vi "Main.vi"(10 "DAQ Type":enum16{"Hardware", "Simulation"}(ring), 11 "Module Admin":refnum<class "Delacor_lib_QMH_Module Admin.lvclass">) -> ()   [LabVIEW 2021, in "CVT.lvlib"]
doc: "This template is based off of the Queued Message Handler design pattern and the Queued Message Handler project template that ships with LabVIEW.\n\nThe main difference is that the queue is private to this module and communication between modules is performed via Broadcast and Request events.\n\nRequest events are wrapped in public API methods and are handled in the Event Handling Loop (EHL) of this VI. Any module can register for Broadcast events sent by this module. The EHL generates messages based on user interface actions.\n\nThe Message Handling Loop (MHL) processes messages generated by the EHL, or by other messages. The messages are string values, so new messages can be added easily to the Message Cases case structure in the MHL. Each message cluster can also provide an optional value for Message Data, which is a variant that can be converted to whatever message-specific data is required.\n_____\nBased on DQMH Project Template 6.1.0.94."
uses:
  CVT.lvlib
  <vilib>/Delacor/Delacor QMH/Libraries/Module Admin_class/Delacor_lib_QMH_Module Admin.lvclass
  <vilib>/NI/Current Value Table/Type Defs/File Format.ctl
  <vilib>/NI/Current Value Table/Type Defs/Single Tag.ctl
  <vilib>/NI/Current Value Table/Type Defs/Data Types.ctl
  <vilib>/NI/Current Value Table/Type Defs/Tag Grouping set.ctl
  Module Data--cluster.ctl
  <vilib>/Delacor/Delacor QMH/Libraries/Message Queue_class/Delacor_lib_QMH_Message Queue.lvclass/Delacor_lib_QMH_Message Queue.ctl
  Stop Argument--cluster.ctl
  <vilib>/Delacor/Delacor QMH/Libraries/Module Admin_class/Delacor_lib_QMH_Module Admin.lvclass/Delacor_lib_QMH_Module Admin.ctl
  REQ DC PWS Connect Argument--cluster.ctl
  Input Command.ctl
  REQ Write AO Data Argument--cluster.ctl
  <vilib>/Utility/miscctls.llb/LVPointTypeDef.ctl
  <vilib>/NI/Current Value Table/Type Defs/Group Data.ctl
  <vilib>/Delacor/Delacor QMH/Libraries/Message Queue_class/Delacor_lib_QMH_Enqueue Message (Single).vi
  <vilib>/Delacor/Delacor QMH/Libraries/Module Admin_class/Delacor_lib_QMH_Get External Launch.vi
  <vilib>/NI/Current Value Table/DataTypes/Boolean_Write.vi
  <vilib>/NI/Current Value Table/DataTypes/Double_Get Index.vi
  <vilib>/NI/Current Value Table/Type to Enum.vi
  <vilib>/NI/Current Value Table/DataTypes/Boolean_Type To Enum.vi
  <vilib>/NI/Current Value Table/DataTypes/Double_Type To Enum.vi
  <vilib>/NI/Current Value Table/Read tags into grouped data.vi
  <vilib>/NI/Current Value Table/Write grouped data to tags.vi
  <vilib>/NI/Current Value Table/Read Index Set.vi
  <vilib>/NI/Current Value Table/DataTypes/Double_Read Index Set.vi
  <vilib>/NI/Current Value Table/DataTypes/Array of String_Read Index Set.vi
  <vilib>/NI/Current Value Table/DataTypes/Array of Boolean_Read Index Set.vi
  <vilib>/NI/Current Value Table/DataTypes/Array of Single_Read Index Set.vi
  <vilib>/NI/Current Value Table/DataTypes/Array of Double_Read Index Set.vi
  <vilib>/NI/Current Value Table/DataTypes/Array of I8_Read Index Set.vi
  <vilib>/NI/Current Value Table/DataTypes/Array of I16_Read Index Set.vi
  <vilib>/NI/Current Value Table/DataTypes/Array of I32_Read Index Set.vi
  <vilib>/NI/Current Value Table/DataTypes/Array of I64_Read Index Set.vi
  <vilib>/NI/Current Value Table/DataTypes/Array of U64_Read Index Set.vi
  <vilib>/NI/Current Value Table/DataTypes/Array of U32_Read Index Set.vi
  <vilib>/NI/Current Value Table/DataTypes/Array of U16_Read Index Set.vi
  <vilib>/NI/Current Value Table/DataTypes/Array of U8_Read Index Set.vi
  <vilib>/NI/Current Value Table/DataTypes/Boolean_Read Index Set.vi
  <vilib>/NI/Current Value Table/DataTypes/String_Read Index Set.vi
  <vilib>/NI/Current Value Table/DataTypes/U8_Read Index Set.vi
  <vilib>/NI/Current Value Table/DataTypes/U16_Read Index Set.vi
  <vilib>/NI/Current Value Table/DataTypes/U32_Read Index Set.vi
  <vilib>/NI/Current Value Table/DataTypes/U64_Read Index Set.vi
  <vilib>/NI/Current Value Table/DataTypes/I8_Read Index Set.vi
  <vilib>/NI/Current Value Table/DataTypes/I16_Read Index Set.vi
  <vilib>/NI/Current Value Table/DataTypes/I32_Read Index Set.vi
  <vilib>/NI/Current Value Table/DataTypes/I64_Read Index Set.vi
  <vilib>/NI/Current Value Table/DataTypes/Single_Read Index Set.vi
  <vilib>/NI/Current Value Table/Write Index Set.vi
  <vilib>/NI/Current Value Table/DataTypes/Double_Write Index Set.vi
  <vilib>/NI/Current Value Table/DataTypes/Array of String_Write Index Set.vi
  <vilib>/NI/Current Value Table/DataTypes/Array of Boolean_Write Index Set.vi
  <vilib>/NI/Current Value Table/DataTypes/Array of Single_Write Index Set.vi
  <vilib>/NI/Current Value Table/DataTypes/Array of Double_Write Index Set.vi
  <vilib>/NI/Current Value Table/DataTypes/Array of I8_Write Index Set.vi
  <vilib>/NI/Current Value Table/DataTypes/Array of I16_Write Index Set.vi
  <vilib>/NI/Current Value Table/DataTypes/Array of I32_Write Index Set.vi
  <vilib>/NI/Current Value Table/DataTypes/Array of I64_Write Index Set.vi
  <vilib>/NI/Current Value Table/DataTypes/Array of U64_Write Index Set.vi
  <vilib>/NI/Current Value Table/DataTypes/Array of U32_Write Index Set.vi
  <vilib>/NI/Current Value Table/DataTypes/Array of U16_Write Index Set.vi
  <vilib>/NI/Current Value Table/DataTypes/Array of U8_Write Index Set.vi
  <vilib>/NI/Current Value Table/DataTypes/Boolean_Write Index Set.vi
  <vilib>/NI/Current Value Table/DataTypes/String_Write Index Set.vi
  <vilib>/NI/Current Value Table/DataTypes/U8_Write Index Set.vi
  <vilib>/NI/Current Value Table/DataTypes/U16_Write Index Set.vi
  <vilib>/NI/Current Value Table/DataTypes/U32_Write Index Set.vi
  <vilib>/NI/Current Value Table/DataTypes/U64_Write Index Set.vi
  <vilib>/NI/Current Value Table/DataTypes/I8_Write Index Set.vi
  <vilib>/NI/Current Value Table/DataTypes/I16_Write Index Set.vi
  <vilib>/NI/Current Value Table/DataTypes/I32_Write Index Set.vi
  <vilib>/NI/Current Value Table/DataTypes/I64_Write Index Set.vi
  <vilib>/NI/Current Value Table/DataTypes/Single_Write Index Set.vi
  <vilib>/Utility/error.llb/Error Cluster From Error Code.vi
  <vilib>/NI/Current Value Table/FGVs/CVT Globals.vi
  <vilib>/NI/Current Value Table/FGVs/Tag Memory.vi
  <vilib>/NI/Current Value Table/Memory Block.vi
  <vilib>/NI/Current Value Table/DataTypes/Boolean_Memory Block.vi
  <vilib>/NI/Current Value Table/FGVs/Group Memory.vi
  <vilib>/NI/Current Value Table/DataTypes/Double_Memory Block.vi
  <vilib>/NI/Current Value Table/DataTypes/Array of String_Memory Block.vi
  <vilib>/NI/Current Value Table/DataTypes/Array of Boolean_Memory Block.vi
  <vilib>/NI/Current Value Table/DataTypes/Array of Single_Memory Block.vi
  <vilib>/NI/Current Value Table/DataTypes/Array of Double_Memory Block.vi
  <vilib>/NI/Current Value Table/DataTypes/Array of I8_Memory Block.vi
  <vilib>/NI/Current Value Table/DataTypes/Array of I16_Memory Block.vi
  <vilib>/NI/Current Value Table/DataTypes/Array of I32_Memory Block.vi
  <vilib>/NI/Current Value Table/DataTypes/Array of I64_Memory Block.vi
  <vilib>/NI/Current Value Table/DataTypes/Array of U64_Memory Block.vi
  <vilib>/NI/Current Value Table/DataTypes/Array of U32_Memory Block.vi
  <vilib>/NI/Current Value Table/DataTypes/Array of U16_Memory Block.vi
  <vilib>/NI/Current Value Table/DataTypes/Array of U8_Memory Block.vi
  <vilib>/NI/Current Value Table/DataTypes/String_Memory Block.vi
  <vilib>/NI/Current Value Table/DataTypes/U8_Memory Block.vi
  <vilib>/NI/Current Value Table/DataTypes/U16_Memory Block.vi
  <vilib>/NI/Current Value Table/DataTypes/U32_Memory Block.vi
  <vilib>/NI/Current Value Table/DataTypes/U64_Memory Block.vi
  <vilib>/NI/Current Value Table/DataTypes/I8_Memory Block.vi
  <vilib>/NI/Current Value Table/DataTypes/I16_Memory Block.vi
  <vilib>/NI/Current Value Table/DataTypes/I32_Memory Block.vi
  <vilib>/NI/Current Value Table/DataTypes/I64_Memory Block.vi
  <vilib>/NI/Current Value Table/DataTypes/Single_Memory Block.vi
  <vilib>/ErrorRing/Error Ring.xnode
  <vilib>/Delacor/Delacor QMH/Libraries/Message Queue_class/Delacor_lib_QMH_Message Queue.lvclass
  DAQ Hardware/DAQ Hardware.lvlib
  Error Log/Error Log.lvlib
  <vilib>/NI/Current Value Table/Current Value Table.lvlib
panel:
  out "CVT Tags to Create Out":T1
  in  "CVT Tags to Create":T1
  out "error out":errorcluster
  out "Status":string
  in  "Simulate MHL Error":bool
  in  "Simulate EHL Error":bool
  # "Other QMH Modules communicate with this Module via its Public API (wrappers for its Request Events).\n\nThis Module communicates with other Modules via its Broadcast Events.\nAny module that wants to get these messages, just registers for this module's Broadcast events."
  # "This template is for the Delacor Modified Queued Message Handler design pattern.\n\nSee the block diagram for more information on how to use this template."
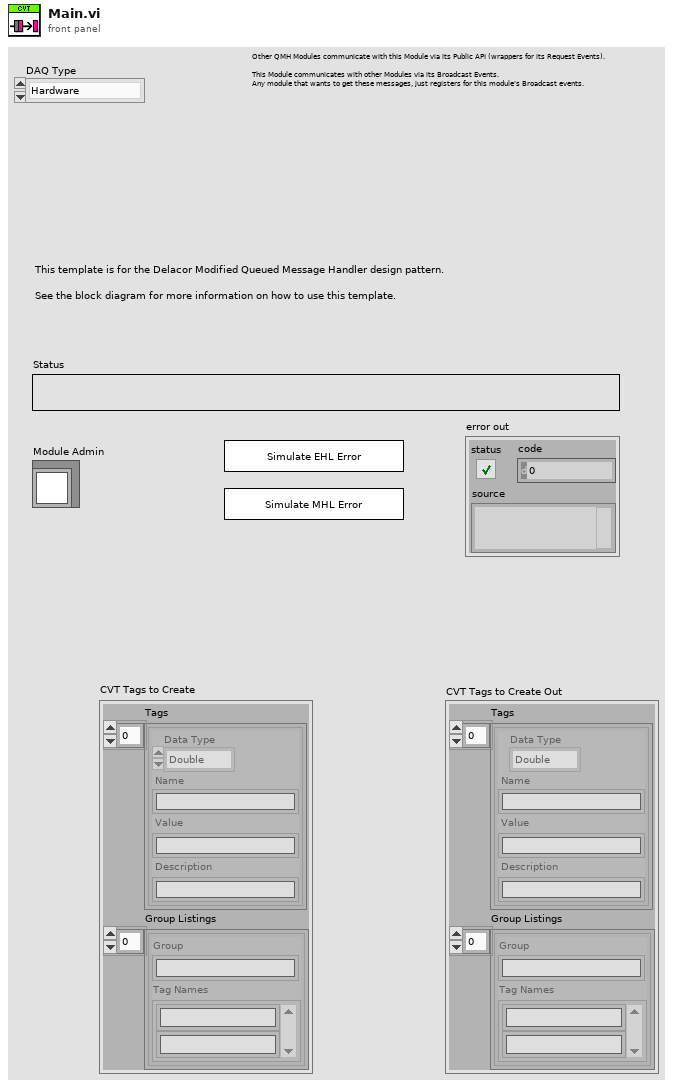
[diagram p1: front panel]
types:
  T1 = typedef "Current Value Table.lvlib/File Format.ctl" = cluster{"Tags":T2[], "Group Listings":T4[]}
  T2 = typedef "Current Value Table.lvlib/Single Tag.ctl" = cluster{"Data Type":T3, "Name":string, "Value":string, "Description":string}
  T3 = typedef "Current Value Table.lvlib/Data Types.ctl" = enum16{"Double", "Single", "I64", "I32", "I16", "I8", "U64", "U32", "U16", "U8", "String", "Boolean", "Array of U8", "Array of U16", "Array of U32", "Array of U64", "Array of I64", "Array of I32", "Array of I16", "Array of I8", "Array of Double", "Array of Single", "Array of Boolean", "Array of String"}
  T4 = typedef "Current Value Table.lvlib/Tag Grouping set.ctl" = cluster{"Group":string, "Tag Names":string[]}
  T5 = typedef "CVT.lvlib/Request Events--cluster.ctl" = cluster{"Stop Module":refnum<user-event>, "Show Panel":refnum<user-event>, "Hide Panel":refnum<user-event>, "Get Module Execution Status":refnum<user-event>, "Show Diagram":refnum<user-event>, "REQ DC PWS Connect":refnum<user-event>, "REQ Write AO Data":refnum<user-event>}
  T6 = typedef "CVT.lvlib/Module Data--cluster.ctl" = cluster{"Status":string}
  T7 = enum32{"invalid lock state", "Not Locked", "Locked (No Password)", "Password-protected"}
  T8 = typedef "CVT.lvlib/Stop Argument--cluster.ctl" = cluster{"Origin":string, "Exit via Stop Module Req?":bool, "Wait for Module to stop?":bool}
  T9 = typedef "CVT.lvlib/REQ DC PWS Connect Argument--cluster.ctl" = cluster{"Connect ?":bool, "Command":T10}
  T10 = typedef "CVT.lvlib/Input Command.ctl" = enum16{"DC PWS", "DMM", "FGEN", "Oscill", "NI DAQ", "NI DIO", "NI CAN", "ESPEC", "ARINC", "MATRIX"}
  T11 = typedef "CVT.lvlib/REQ Write AO Data Argument--cluster.ctl" = cluster{"AO Name":string, "Data":dbl}
  T12 = typedef "LVPointTypeDef.ctl" = cluster{"Horizontal":i16, "Vertical":i16}
  T13 = enum32{"Invalid", "Standard", "Closed", "Hidden", "Minimized", "Maximized"}
  T14 = typedef "Current Value Table.lvlib/Group Data.ctl" = cluster{"Double":dbl[], "Single":sgl[], "I64":i64[], "I32":i32[], "I16":i16[], "I8":i8[], "U64":u64[], "U32":u32[], "U16":u16[], "U8":u8[], "String":string[], "Boolean":bool[], "Array of U8":cluster{"U8 Array":u8[]}[], "Array of U16":cluster{"U16 Array":u16[]}[], "Array of U32":cluster{"U32 Array":u32[]}[], "Array of U64":cluster{"U64 Array":u64[]}[], "Array of I64":cluster{"I64 Array":i64[]}[], "Array of I32":cluster{"I32 Array":i32[]}[], "Array of I16":cluster{"I16 Array":i16[]}[], "Array of I8":cluster{"I8 Array":i8[]}[], "Array of Double":cluster{"DBL Array":dbl[]}[], "Array of Single":cluster{"SGL Array":sgl[]}[], "Array of Boolean":cluster{"Boolean Array":bool[]}[], "Array of String":cluster{"String Array":string[]}[]}
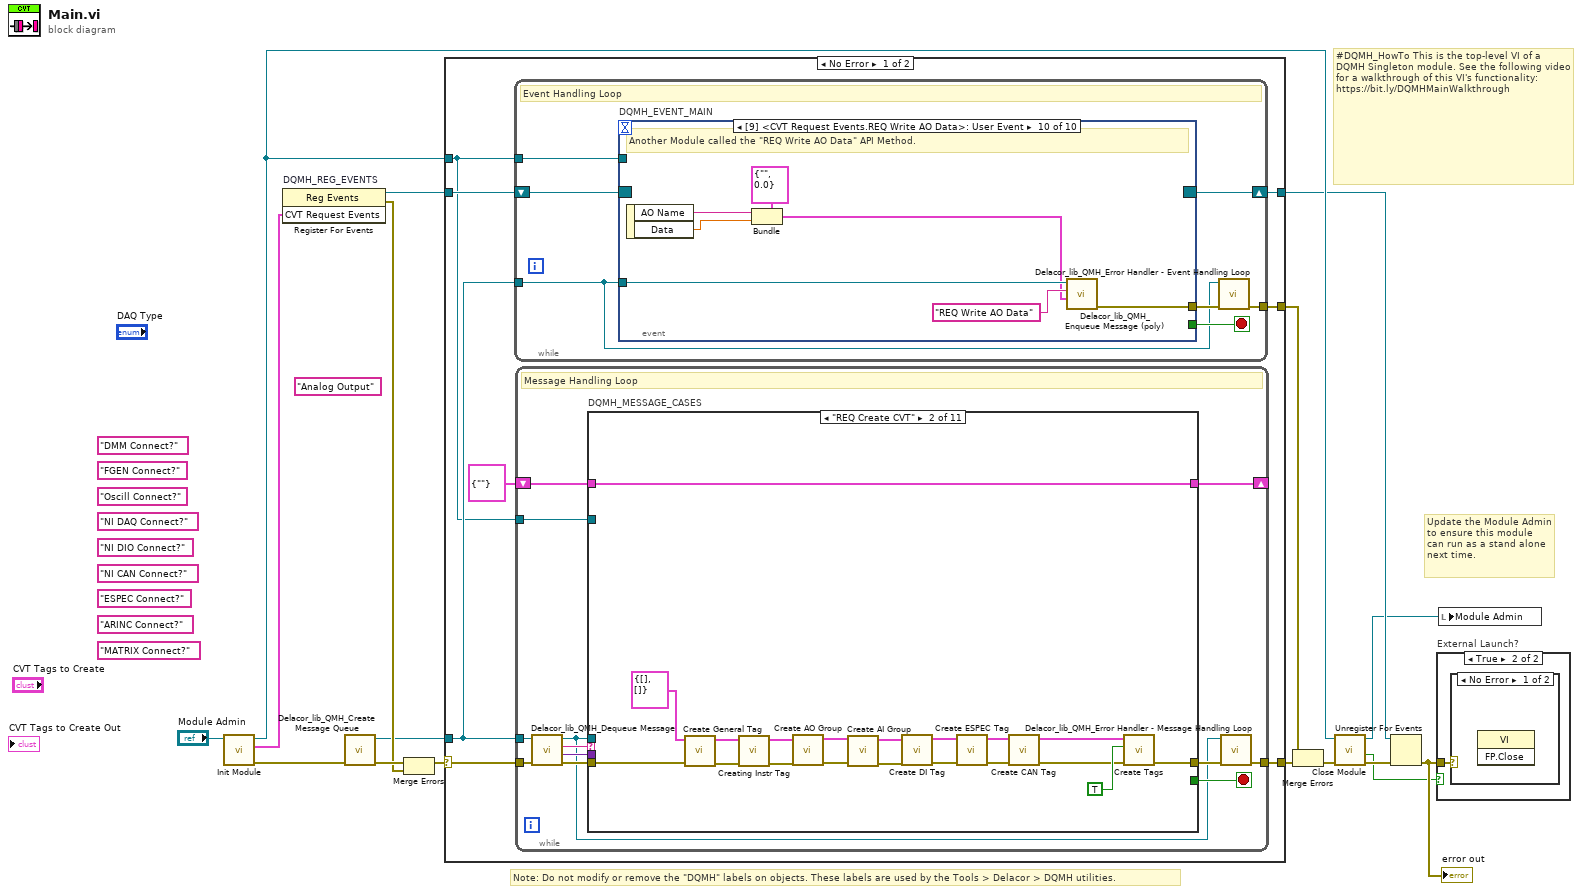
[diagram p0: block diagram]
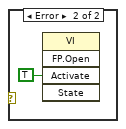
[diagram p3: hidden frame]
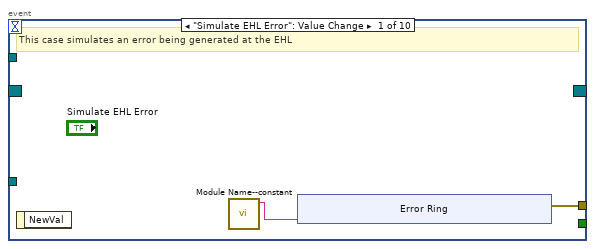
[diagram p4: hidden frame]
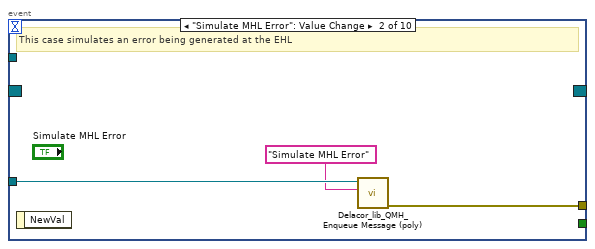
[diagram p5: hidden frame]
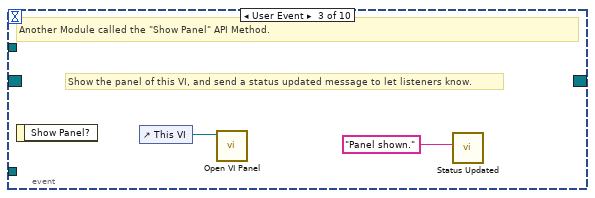
[diagram p6: hidden frame]
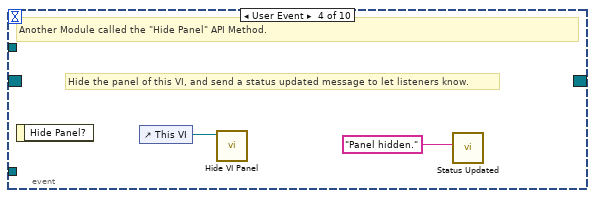
[diagram p7: hidden frame]
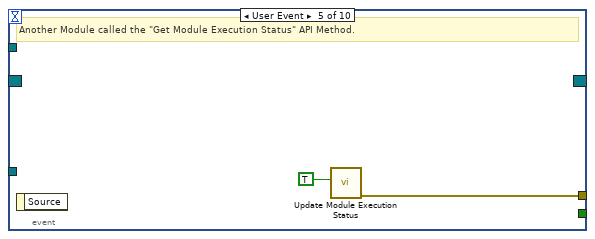
[diagram p8: hidden frame]
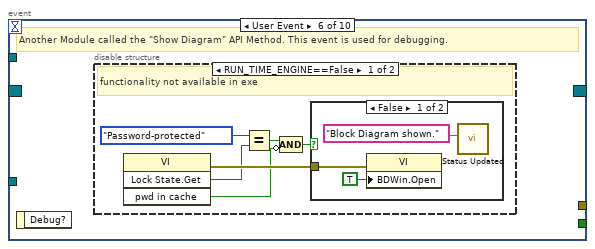
[diagram p9: hidden frame]
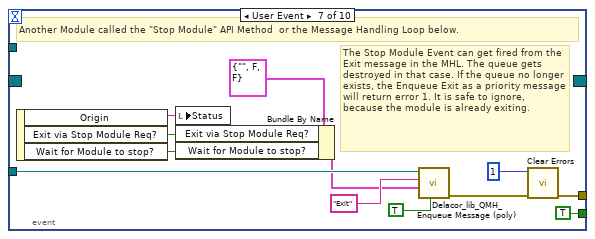
[diagram p12: hidden frame]
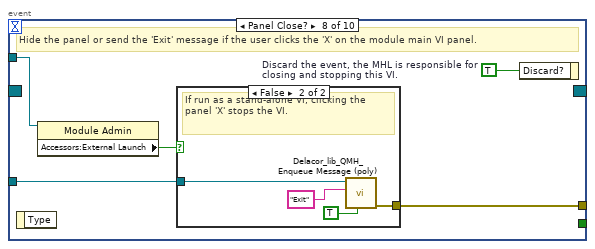
[diagram p13: hidden frame]
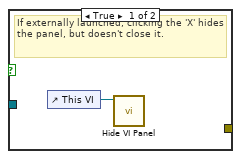
[diagram p14: hidden frame]
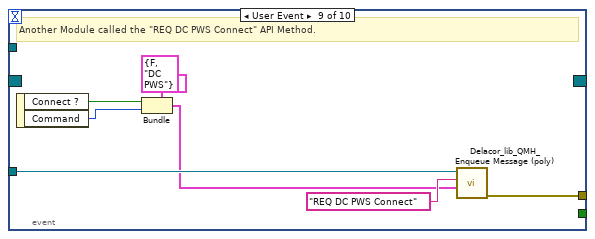
[diagram p15: hidden frame]
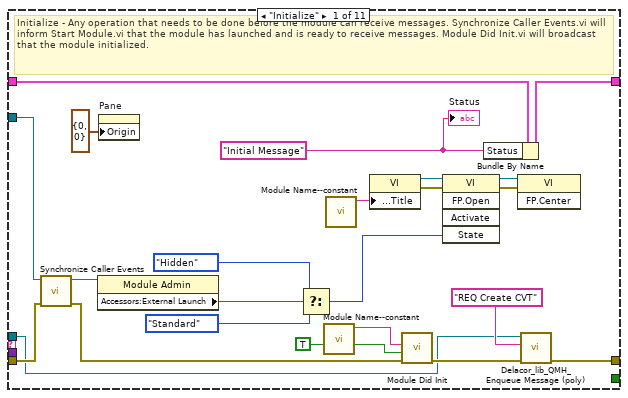
[diagram p16: hidden frame]
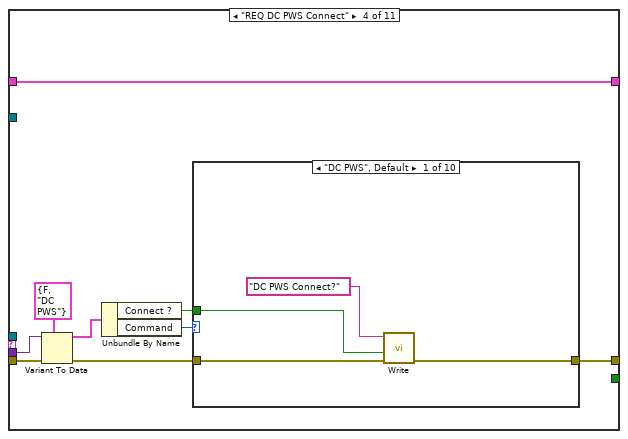
[diagram p18: hidden frame]
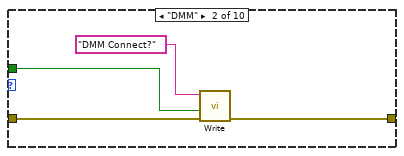
[diagram p19: hidden frame]
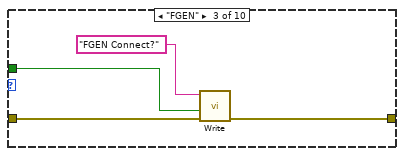
[diagram p20: hidden frame]
diagram:
  (unwired) "Analog Output" ("Group")
  (unwired) "MATRIX Connect?" ("Tag Name")
  (unwired) "ARINC Connect?" ("Tag Name")
  (unwired) "ESPEC Connect?" ("Tag Name")
  (unwired) "NI CAN Connect?" ("Tag Name")
  (unwired) "NI DIO Connect?" ("Tag Name")
  (unwired) "NI DAQ Connect?" ("Tag Name")
  (unwired) "Oscill Connect?" ("Tag Name")
  (unwired) "FGEN Connect?" ("Tag Name")
  (unwired) "DMM Connect?" ("Tag Name")
  # "#DQMH_HowTo This is the top-level VI of a DQMH Singleton module. See the following video for a walkthrough of this VI's functionality: https://bit.ly/DQMHMainWalkthrough"
  # "Note: Do not modify or remove the \"DQMH\" labels on objects. These labels are used by the Tools > Delacor > DQMH utilities."
  # "Update the Module Admin to ensure this module can run as a stand alone next time."
  n1 = call "Init Module.vi"("Singleton Module Admin in"="Module Admin") -> ("error out"=w16:errorcluster, "CVT Request Events"=w5:T5, "Singleton Module Admin out"=w8:refnum<class "Delacor_lib_QMH_Module Admin.lvclass">)  [unwired: 8 in]
  n2 = register-events "DQMH_REG_EVENTS"(w5) -> (reference out=w6:refnum<event-registration>, error out=w9:errorcluster)  [unwired: 2 in]
  n3 = call <vilib>:"Delacor_lib_QMH_Create Message Queue.vi"("error in"=w16) -> ("error out"=w11:errorcluster, "Message Queue"=w4:refnum<class "Delacor_lib_QMH_Message Queue.lvclass">)  [unwired: 9 in]
  n4 = Merge Errors(w11, w9) -> (w10:errorcluster)
  n5 = case shown="No Error" w10 {
    selector: w10 -> [w23 w286]
    tunnel: [w25 w285] -> w17
    tunnel: [w22 w291] -> w7
    tunnel: w6 -> [w20 w291]
    tunnel: w4 -> [w19 w284]
    tunnel: [w24 _] -> w14
    tunnel: w8 -> [w18 w287]
    frame No Error {
      n6 = while {
        tunnel: w19 -> [w26]
        shift-right: [w29] -> w22
        shift-left: w20 -> [w30]
        tunnel: [w31] -> w24
        tunnel: w18 -> [w27]
        stop <- w28 stop-if-true
        # "Event Handling Loop"
        n7 = event "DQMH_EVENT_MAIN" shown="[9] <CVT Request Events.REQ Write AO Data>: User Event" {
          selector: w30 -> [_ _ _ _ _ _ _ _ _ _]
          dyn-events: [_ _ _ _ _ _ _ _ _ _] -> w29
          timeout: _ -> [_ _ _ _ _ _ _ _ _ _]
          tunnel: [_ _ _ _ _ _ TRUE ("Discard?") _ _ _] -> w28
          tunnel: w26 -> [_ w43 _ _ _ _ w67 w74 w88 w95]
          tunnel: [w34 w44 _ _ w50 _ w70 w76 w83 w91] -> w32
          tunnel: w27 -> [_ _ _ _ _ _ _ w73 _ _]
          event "Simulate EHL Error": Value Change {
            # "This case simulates an error being generated at the EHL"
            n8 = event-data() -> ()  [unwired: 1 in, 1 out]
            n9 = call "Module Name--constant.vi"() -> ("Module Name"=w33:string)  [unwired: 11 in]
            n10 = xnode "Error Ring"("parameter 0"=w33) -> ("error out"=w34:errorcluster)
          }
          event "Simulate MHL Error": Value Change {
            # "This case simulates an error being generated at the EHL"
            n11 = event-data() -> ()  [unwired: 1 in, 1 out]
            n12 = call-poly <vilib>:"Delacor_lib_QMH_Enqueue Message (poly).vi"("Message"="Simulate MHL Error", "Message Queue in"=w43) -> ("error out"=w44:errorcluster)  [unwired: 8 in, 1 out]
          }
          event User Event {
            # "Show the panel of this VI, and send a status updated message to let listeners know."
            # "Another Module called the \"Show Panel\" API Method."
            n13 = event-data() -> ()  [unwired: 1 in, 1 out]
            n14 = control-ref of="This VI"() -> (w46:refnum<vi>)
            n15 = call "Open VI Panel.vi"("VI"=w46) -> ()  [unwired: 10 in, 1 out]
            n16 = call "Status Updated.vi"("Status"="Panel shown." ("format string")) -> ()  [unwired: 10 in, 1 out]
          }
          event User Event {
            # "Hide the panel of this VI, and send a status updated message to let listeners know."
            # "Another Module called the \"Hide Panel\" API Method."
            n17 = event-data() -> ()  [unwired: 1 in, 1 out]
            n18 = control-ref of="This VI"() -> (w48:refnum<vi>)
            n19 = call "Hide VI Panel.vi"("VI"=w48) -> ()  [unwired: 10 in, 1 out]
            n20 = call "Status Updated.vi"("Status"="Panel hidden." ("format string")) -> ()  [unwired: 10 in, 1 out]
          }
          event User Event {
            # "Another Module called the \"Get Module Execution Status\" API Method."
            n21 = event-data() -> ()  [unwired: 1 in, 1 out]
            n22 = call "Update Module Execution Status.vi"("Running?"=TRUE) -> ("error out"=w50:errorcluster)  [unwired: 10 in]
          }
          event User Event {
            # "Another Module called the \"Show Diagram\" API Method. This event is used for debugging."
            n23 = event-data() -> ()  [unwired: 1 in, 1 out]
            n24 = disable-structure shown="RUN_TIME_ENGINE==False" {
              frame condition #0 (active) {
                # "functionality not available in exe"
                n25 = invoke class="VI" method="Lock State.Get"() -> (error out=w56:errorcluster, "Get Lock State"=w55:T7, "pwd in cache"=w52:bool)  [unwired: 4 in, 1 out]
                n26 = Equal?(x=T7."Password-protected", y=w55) -> (x = y?=w53:bool)
                n27 = Compound Arithmetic op=AND(w53, invert w52) -> (w51:bool)
                n28 = case shown="False" w51 {
                  tunnel: w56 -> [w59 _]
                  frame False {
                    n29 = property class="VI"(error in=w59, "BDWin.Open"=TRUE ("Block Diagram Window:Open")) -> ()  [unwired: 1 in, 2 out]
                    n30 = call "Status Updated.vi"("Status"="Block Diagram shown." ("format string")) -> ()  [unwired: 10 in, 1 out]
                  }
                  frame True {
                    # "Password-protected VI, and the password is not in the cache. Do not show the diagram."
                  }
                }
              }
              frame condition #1 {
              }
            }
          }
          event User Event {
            # "The Stop Module Event can get fired from the Exit message in the MHL. The queue gets destroyed in that case. If the queue no longer exists, the Enqueue Exit as a priority message will return error 1. It is safe to ignore, because the module is already exiting."
            # "Another Module called the \"Stop Module\" API Method  or the Message Handling Loop below."
            n31 = event-data() -> ("Origin"=w66:string, "Exit via Stop Module Req?"=w62:bool, "Wait for Module to stop?"=w61:bool)  [unwired: 1 in]
            n32 = local write "Status"(w66) -> ()
            n33 = Bundle By Name(cluster=T8 {"Origin"="", "Exit via Stop Module Req?"=FALSE, "Wait for Module to stop?"=FALSE} ("Stop Argument"), "Exit via Stop Module Req?"=w62, "Wait for Module to stop?"=w61) -> (w60:T8)
            n34 = call-poly <vilib>:"Delacor_lib_QMH_Enqueue Message (poly).vi"("Priority Message? (F)"=TRUE, "Message Data"=w60, "Message"="Exit", "Message Queue in"=w67) -> ("error out"=w71:errorcluster)  [unwired: 6 in, 1 out]
            n35 = call <vilib>:"Clear Errors.vi"("error in (no error)"=w71, "specific error code to clear (0: all)"=1) -> ("error out"=w70:errorcluster)  [unwired: 4 in, 1 out]
          }
          event Panel Close? {
            w75 = TRUE  # Discard the event, the MHL is responsible for closing and stopping this VI.
            # "Hide the panel or send the 'Exit' message if the user clicks the 'X' on the module main VI panel."
            n36 = event-data() -> ()  [unwired: 1 in, 1 out]
            n37 = property class="Module Admin"(reference=w73) -> ("Accessors:External Launch"=w72:bool)  [unwired: 1 in, 2 out]
            n38 = case shown="False" w72 {
              tunnel: w74 -> [_ w80]
              tunnel: [_ w81] -> w76
              frame True {
                # "If externally launched, clicking the 'X' hides the panel, but doesn't close it."
                n39 = control-ref of="This VI"() -> (w77:refnum<vi>)
                n40 = call "Hide VI Panel.vi"("VI"=w77) -> ()  [unwired: 10 in, 1 out]
              }
              frame False {
                # "If run as a stand-alone VI, clicking the panel 'X' stops the VI."
                n41 = call-poly <vilib>:"Delacor_lib_QMH_Enqueue Message (poly).vi"("Priority Message? (F)"=TRUE, "Message"="Exit", "Message Queue in"=w80) -> ("error out"=w81:errorcluster)  [unwired: 7 in, 1 out]
              }
            }
            n42 = event-data("Discard?"=w75) -> ()  [unwired: 1 in, 1 out]
          }
          event User Event {
            # "Another Module called the \"REQ DC PWS Connect\" API Method."
            n43 = event-data() -> ("Connect ?"=w84:bool, "Command"=w82:T10)  [unwired: 1 in]
            n44 = Bundle(cluster=T9 {"Connect ?"=FALSE, "Command"=enum."DC PWS"} ("REQ DC PWS Connect Argument"), "Connect ?"=w84, "Command"=w82) -> (w85:T9)
            n45 = call-poly <vilib>:"Delacor_lib_QMH_Enqueue Message (poly).vi"("Message Data"=w85, "Message"="REQ DC PWS Connect", "Message Queue in"=w88) -> ("error out"=w83:errorcluster)  [unwired: 7 in, 1 out]
          }
          event User Event {
            # "Another Module called the \"REQ Write AO Data\" API Method."
            n46 = event-data() -> ("AO Name"=w90:string, "Data"=w89:dbl)  [unwired: 1 in]
            n47 = Bundle(cluster=T11 {"AO Name"="", "Data"=0.0} ("REQ Write AO Data Argument"), "AO Name"=w90, "Data"=w89) -> (w92:T11)
            n48 = call-poly <vilib>:"Delacor_lib_QMH_Enqueue Message (poly).vi"("Message Data"=w92, "Message"="REQ Write AO Data", "Message Queue in"=w95) -> ("error out"=w91:errorcluster)  [unwired: 7 in, 1 out]
          }
        }
        n49 = call-dynamic "Delacor_lib_QMH_Error Handler - Event Handling Loop.vi"("error in"=w32, "Message Queue in"=w26) -> ("dup error in"=w31:errorcluster)  [unwired: 8 in, 1 out]
      }
      n50 = while {
        tunnel: w19 -> [w98]
        shift-right: [w102] -> _
        shift-left: T6 {"Status"=""} ("Data Cluster") -> [w103]
        tunnel: w23 -> [w106]
        tunnel: [w104] -> w25
        tunnel: w18 -> [w96]
        stop <- w101 stop-if-true
        # "Message Handling Loop"
        n51 = call-dynamic "Delacor_lib_QMH_Dequeue Message.vi"("error in"=w106, "Message Queue in"=w98) -> ("error out"=w105:errorcluster, "Message Data"=w99:variant, "Message"=w100:string, "Message Queue out"=w97:refnum<class "Delacor_lib_QMH_Message Queue.lvclass">)  [unwired: 6 in]
        n52 = case "DQMH_MESSAGE_CASES" shown="\"REQ Create CVT\"" w100 {
          selector: w100 -> [_ _ _ _ _ _ _ _ _ _ w271]
          tunnel: w97 -> [w108 _ _ _ _ _ _ _ w241 w263 _]
          tunnel: w105 -> [w128 w142 w151 w160 w220 w223 w225 w230 w248 w269 w273]
          tunnel: [w109 w148 w151 w154 w216 w222 w225 w229 w244 w266 w274] -> w107
          tunnel: w103 -> [w118 w149 w150 w159 w219 w221 w224 w227 w243 w262 w272]
          tunnel: [w117 w149 w150 w159 w219 w221 w224 w227 w243 w262 w272] -> w102
          tunnel: [_ _ _ _ _ _ _ _ _ w261 _] -> w101
          tunnel: w99 -> [_ _ _ w158 w218 _ _ _ w242 w260 _]
          tunnel: w96 -> [w119 _ _ _ _ _ _ _ w240 w255 _]
          frame "Initialize" {
            w113 = "Initial Message" ("Initial Message")
            # "Initialize - Any operation that needs to be done before the module can receive messages. Synchronize Caller Events.vi will inform Start Module.vi that the module has launched and is ready to receive messages. Module Did Init.vi will broadcast that the module initialized."
            n53 = call "Synchronize Caller Events.vi"("error in (no error)"=w128, "Singleton Module Admin in"=w119) -> ("error out"=w127:errorcluster, "Singleton Module Admin out"=w114:refnum<class "Delacor_lib_QMH_Module Admin.lvclass">)  [unwired: 8 in]
            n54 = property class="Module Admin"(reference=w114) -> ("Accessors:External Launch"=w123:bool)  [unwired: 1 in, 2 out]
            n55 = property on="Pane" class="Pane"("Origin"=T12 {"Horizontal"=0, "Vertical"=0}) -> ()  [unwired: 2 in, 2 out]
            n56 = Select(t=T13."Hidden" ("State"), s=w123, f=T13."Standard" ("State")) -> (s? t:f=w120:T13)
            n57 = call "Module Name--constant.vi"() -> ("Module Name"=w115:string)  [unwired: 11 in]
            n58 = call "Module Name--constant.vi"() -> ("Module Name"=w126:string)  [unwired: 11 in]
            n59 = property class="VI"("Front Panel.Title"=w126) -> (reference out=w125:refnum<vi>, error out=w130:errorcluster)  [unwired: 2 in]
            n60 = call "Module Did Init.vi"("error in (no error)"=w127, "Initialized?"=TRUE, "Origin"=w115) -> ("error out"=w110:errorcluster)  [unwired: 8 in]
            n61 = invoke class="VI" method="FP.Open"(reference=w125, error in=w130, "State"=w120) -> (reference out=w124:refnum<vi>, error out=w129:errorcluster)  [unwired: 2 in, 3 out]
            n62 = Bundle By Name(cluster=w118, "Status"=w113) -> (w117:T6)
            n63 = invoke class="VI" method="FP.Center"(reference=w124, error in=w129) -> ()  [unwired: 1 in, 3 out]
            n64 = call-poly <vilib>:"Delacor_lib_QMH_Enqueue Message (poly).vi"("error in"=w110, "Message"="REQ Create CVT", "Message Queue in"=w108) -> ("error out"=w109:errorcluster)  [unwired: 7 in, 1 out]
            "Status" <- w113
          }
          frame "REQ Create CVT" {
            n65 = call "Create General Tag.vi"("error in (no error)"=w142, "CVT Tags to Create"=T1 {"Tags"=[], "Group Listings"=[]}) -> ("error out"=w140:errorcluster, "CVT Tags to Create Out"=w141:T1)  [unwired: 8 in]
            n66 = call "Creating Instr Tag.vi"("error in (no error)"=w140, "CVT Tags to Create"=w141) -> ("error out"=w139:errorcluster, "CVT Tags to Create Out"=w138:T1)  [unwired: 8 in]
            n67 = call "Create AO Group.vi"("error in (no error)"=w139, "CVT Tags to Create"=w138) -> ("error out"=w146:errorcluster, "CVT Tags to Create Out"=w145:T1)  [unwired: 8 in]
            n68 = call "Create AI Group.vi"("error in (no error)"=w146, "CVT Tags to Create"=w145) -> ("error out"=w144:errorcluster, "CVT Tags to Create Out"=w143:T1)  [unwired: 8 in]
            n69 = call "Create DI Tag.vi"("error in (no error)"=w144, "CVT Tags to Create"=w143) -> ("error out"=w137:errorcluster, "CVT Tags to Create Out"=w136:T1)  [unwired: 8 in]
            n70 = call "Create ESPEC Tag.vi"("error in (no error)"=w137, "CVT Tags to Create"=w136) -> ("error out"=w134:errorcluster, "CVT Tags to Create Out"=w133:T1)  [unwired: 8 in]
            n71 = call "Create CAN Tag.vi"("error in (no error)"=w134, "CVT Tags to Create"=w133) -> ("error out"=w131:errorcluster, "CVT Tags to Create Out"=w132:T1)  [unwired: 8 in]
            n72 = call <vilib>:"Create Tags.vi"("error in (no error)"=w131, "Clear Table? (F)"=TRUE, "CVT Tags to Create"=w132) -> ("error out"=w148:errorcluster)  [unwired: 8 in]
          }
          frame "---Module Specific---" {
            # "Separator -- The following cases handle messages specific to this Module."
          }
          frame "REQ DC PWS Connect" {
            n73 = Variant To Data(error in=w160, type=T9 {"Connect ?"=FALSE, "Command"=enum."DC PWS"} ("REQ DC PWS Connect Argument"), Variant=w158) -> (data=w156:T9, error out=w155:errorcluster)
            n74 = Unbundle By Name(w156) -> ("Connect ?"=w152:bool, "Command"=w153:T10)
            n75 = case shown="\"DC PWS\", Default" w153 {
              tunnel: w155 -> [w164 w168 w172 w176 w180 w184 w188 w192 w196 w200]
              tunnel: [w163 w167 w171 w175 w179 w183 w187 w191 w195 w199] -> w154
              tunnel: w152 -> [w161 w165 w169 w173 w177 w181 w185 w189 w193 w197]
              frame "DC PWS", Default {
                n76 = call-poly <vilib>:"Write.vi"("error in (no error)"=w164, "Value"=w161, "Tag Name"="DC PWS Connect?") -> ("error out"=w163:errorcluster)  [unwired: 8 in]
              }
              frame "DMM" {
                n77 = call-poly <vilib>:"Write.vi"("error in (no error)"=w168, "Value"=w165, "Tag Name"="DMM Connect?") -> ("error out"=w167:errorcluster)  [unwired: 8 in]
              }
              frame "FGEN" {
                n78 = call-poly <vilib>:"Write.vi"("error in (no error)"=w172, "Value"=w169, "Tag Name"="FGEN Connect?") -> ("error out"=w171:errorcluster)  [unwired: 8 in]
              }
              frame "Oscill" {
                n79 = call-poly <vilib>:"Write.vi"("error in (no error)"=w176, "Value"=w173, "Tag Name"="Oscill Connect?") -> ("error out"=w175:errorcluster)  [unwired: 8 in]
              }
              frame "NI DAQ" {
                n80 = call-poly <vilib>:"Write.vi"("error in (no error)"=w180, "Value"=w177, "Tag Name"="NI DAQ Connect?") -> ("error out"=w179:errorcluster)  [unwired: 8 in]
              }
              frame "NI DIO" {
                n81 = call-poly <vilib>:"Write.vi"("error in (no error)"=w184, "Value"=w181, "Tag Name"="NI DIO Connect?") -> ("error out"=w183:errorcluster)  [unwired: 8 in]
              }
              frame "NI CAN" {
                n82 = call-poly <vilib>:"Write.vi"("error in (no error)"=w188, "Value"=w185, "Tag Name"="NI CAN Connect?") -> ("error out"=w187:errorcluster)  [unwired: 8 in]
              }
              frame "ESPEC" {
                n83 = call-poly <vilib>:"Write.vi"("error in (no error)"=w192, "Value"=w189, "Tag Name"="ESPEC Connect?") -> ("error out"=w191:errorcluster)  [unwired: 8 in]
              }
              frame "ARINC" {
                n84 = call-poly <vilib>:"Write.vi"("error in (no error)"=w196, "Value"=w193, "Tag Name"="ARINC Connect?") -> ("error out"=w195:errorcluster)  [unwired: 8 in]
              }
              frame "MATRIX" {
                n85 = call-poly <vilib>:"Write.vi"("error in (no error)"=w200, "Value"=w197, "Tag Name"="MATRIX Connect?") -> ("error out"=w199:errorcluster)  [unwired: 8 in]
              }
            }
          }
          frame "REQ Write AO Data" {
            n86 = Variant To Data(error in=w220, type=T11 {"AO Name"="", "Data"=0.0} ("REQ Write AO Data Argument"), Variant=w218) -> (data=w206:T11, error out=w203:errorcluster)
            n87 = Unbundle By Name(w206) -> ("AO Name"=w205:string, "Data"=w204:dbl)
            n88 = call-poly <vilib>:"Get Index.vi"("error in (no error)"=w203, "Tag Name"=w205) -> ("error out"=w215:errorcluster, "Index"=w211:i32)  [unwired: 8 in]
            n89 = call <vilib>:"Read Grouped Tags.vi"("error in (no error)"=w215, "Group"="Analog Output") -> ("error out"=w210:errorcluster, "Data"=w213:T14)  [unwired: 8 in]
            n90 = Unbundle By Name(w213) -> ("Double"=w212:dbl[])
            n91 = Replace Array Subset(array=w212, new element=w204, index=w211) -> (w209:dbl[])
            n92 = Bundle By Name(cluster=T14 {"Double"=[], "Single"=[], "I64"=[], "I32"=[], "I16"=[], "I8"=[], "U64"=[], "U32"=[], "U16"=[], "U8"=[], "String"=[], "Boolean"=[], "Array of U8"=[], "Array of U16"=[], "Array of U32"=[], "Array of U64"=[], "Array of I64"=[], "Array of I32"=[], "Array of I16"=[], "Array of I8"=[], "Array of Double"=[], "Array of Single"=[], "Array of Boolean"=[], "Array of String"=[]} ("Data"), "Double"=w209) -> (w207:T14)
            n93 = call <vilib>:"Write Grouped Tags.vi"("error in (no error)"=w210, "Data"=w207, "Group"="Analog Output") -> ("error out"=w202:errorcluster)  [unwired: 8 in]
            n94 = call "REQ Write AO.vi"("error in"=w202) -> ("error out"=w216:errorcluster)  [unwired: 10 in]
          }
          frame "---Copy This Frame---" {
            # "Duplicate this frame when creating new messages.  Change this comment in the duplicated frame to describe this message."
            n95 = Merge Errors(w223) -> (w222:errorcluster)
          }
          frame "---Exit and Error Handling---" {
            # "Separator - The following cases handle errors and exit messages."
          }
          frame "Simulate MHL Error" {
            # "#DQMH_HowTo The 'Simulate MHL Error' button  illustrates how the MHL handles errors. This event is instructional in nature and can be removed."
            # "Simulate an error occurring at the MHL"
            n96 = call "Module Name--constant.vi"() -> ("Module Name"=w226:string)  [unwired: 11 in]
            n97 = xnode "Error Ring"("parameter 0"=w226) -> ("error out"=w228:errorcluster)
            n98 = Merge Errors(w230, w228) -> (w229:errorcluster)
          }
          frame "Error" {
            # "Error - Check the error message data and respond accordingly. This message is sent by the \"Error Handler\" VIs at the end of each loop in this application."
            n99 = property class="Module Admin"(reference=w240) -> ("Accessors:External Launch"=w239:bool)  [unwired: 1 in, 2 out]
            n100 = Variant To Data(error in=w248, type=errorcluster {"status"=FALSE, "code"=0, "source"=""} ("error constant"), Variant=w242) -> (data=w238:errorcluster, error out=w246:errorcluster)
            n101 = call "Error Reported.vi"("Error"=w238) -> ()  [unwired: 10 in, 1 out]
            n102 = call "REQ Log Error.vi"("error in (no error)"=w238) -> ()  [unwired: 10 in, 1 out]
            n103 = case shown="False" w239 {
              tunnel: [w254 _] -> w245
              tunnel: w241 -> [w252 _]
              tunnel: w238 -> [w253 _]
              frame False {
                n104 = call <vilib>:"Simple Error Handler.vi"("error source (\" \")"="REQ Create CVT", "error in (no error)"=w253) -> ()  [unwired: 3 in, 5 out]
                n105 = call-poly <vilib>:"Delacor_lib_QMH_Enqueue Message (poly).vi"("Priority Message? (F)"=TRUE, "Message"="Exit", "Message Queue in"=w252) -> ("error out"=w254:errorcluster)  [unwired: 7 in, 1 out]
              }
              frame True {
              }
            }
            n106 = Merge Errors(w246, w245) -> (w244:errorcluster)
            n107 = local write "error out"(w244) -> ()
          }
          frame "Exit" {
            w259 = 91  # 91: not all Exit messages will have an argument
            w261 = TRUE  # Stop the VI
            # "Release the message queue reference"
            # "Exit - Exit the application."
            n108 = Variant To Data(error in=w269, type=T8 {"Origin"="", "Exit via Stop Module Req?"=FALSE, "Wait for Module to stop?"=FALSE} ("Stop Argument"), Variant=w260) -> (data=w257:T8, error out=w265:errorcluster)
            n109 = call <vilib>:"Clear Errors.vi"("error in (no error)"=w265, "specific error code to clear (0: all)"=w259) -> ("error out"=w268:errorcluster)  [unwired: 4 in, 1 out]
            n110 = call-dynamic "Delacor_lib_QMH_Release Message Queue.vi"("error in"=w268, "Message Queue"=w263) -> ("error out"=w267:errorcluster)  [unwired: 9 in]
            n111 = control-ref of="This VI"() -> (w256:refnum<vi>)
            n112 = call "Handle Exit.vi"("Stop Argument"=w257, "Admin in"=w255, "VI reference"=w256) -> ("error out"=w264:errorcluster)  [unwired: 7 in, 1 out]
            n113 = Merge Errors(w267, w264) -> (w266:errorcluster)
          }
          frame Default {
            # "'Default' case only runs if there is a message that isn't defined in any of the other cases.  Output a programming error."
            n114 = call "Module Name--constant.vi"() -> ("Module Name"=w270:string)  [unwired: 11 in]
            n115 = xnode "Error Ring"("parameter 0"=w271, "parameter 1"=w270) -> ("error out"=w275:errorcluster)
            n116 = Merge Errors(w273, w275) -> (w274:errorcluster)
          }
        }
        n117 = call-dynamic "Delacor_lib_QMH_Error Handler - Message Handling Loop.vi"("error in"=w107, "Message Queue in"=w97) -> ("dup error in"=w104:errorcluster)  [unwired: 8 in, 1 out]
      }
    }
    frame Error {
      # "Synchronize Caller Events.vi will inform Start Module.vi that the module has launched and will let the code calling Start Module.vi register for broadcasts and would permit the caller receive the broadcast that an error occurred at launch time."
      n118 = call-dynamic "Delacor_lib_QMH_Release Message Queue.vi"("error in"=w286, "Message Queue"=w284) -> ("error out"=w285:errorcluster)  [unwired: 9 in]
      n119 = call "Synchronize Caller Events.vi"("Singleton Module Admin in"=w287) -> ("error out"=w292:errorcluster)  [unwired: 9 in, 1 out]
      n120 = call "Module Name--constant.vi"() -> ("Module Name"=w290:string)  [unwired: 11 in]
      n121 = Format Into String(format string="An error occurred during initialization. %s is no longer running.", w290) -> (resulting string=w288:string)  [unwired: 2 in, 1 out]
      n122 = Merge Errors(w285, w292) -> (w293:errorcluster)
      n123 = call "Error Reported.vi"("Additional Information"=w288, "Error"=w293) -> ()  [unwired: 9 in, 1 out]
    }
  }
  n124 = Merge Errors(w14, w17) -> (w13:errorcluster)
  n125 = call "Close Module.vi"("error in (no error)"=w13, "Module Admin in"=w8) -> ("error out"=w15:errorcluster, "External Launch"=w1:bool, "Module Admin out"=w2:refnum<class "Delacor_lib_QMH_Module Admin.lvclass">)  [unwired: 7 in]
  n126 = Unregister For Events(event registration refnum=w7, error in=w15) -> (error out=w12:errorcluster)
  "error out" <- w12
  n127 = case "External Launch?" shown="True" w1 {
    tunnel: w12 -> [_ w294]
    frame False {
    }
    frame True {
      n128 = case shown="No Error" w294 {
        frame No Error {
          n129 = invoke class="VI" method="FP.Close"() -> ()  [unwired: 3 in, 3 out]
        }
        frame Error {
          n130 = invoke class="VI" method="FP.Open"("Activate"=TRUE ("Activate?")) -> ()  [unwired: 4 in, 5 out]
        }
      }
    }
  }
  n131 = local write "Module Admin"(w2) -> ()
